vi "Model Identifyer.vi"(9 "Manufacturer":T1=enum."red", 11 "ID String":string) -> (1 "Result":bool)   [LabVIEW 2014, in "Universal Power Meter.lvlib" / "Universal Power Meter.lvclass"]
uses:
  Universal Power Meter.lvclass
  Manufacturer List.ctl
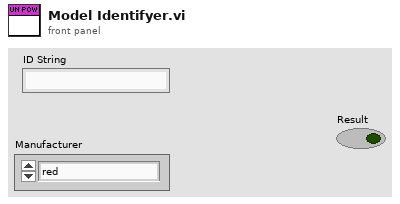
[diagram p1: front panel]
types:
  T1 = typedef "Manufacturer List.ctl" = enum16{"National Instruments", "TEKTRONIX", "FLUKE", "dummy", "red", "YOKOGAWA"}
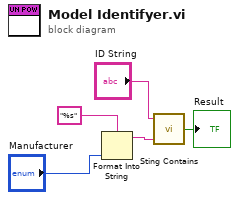
[diagram p0: block diagram]
diagram:
  n1 = Format Into String(format string="%s", "Manufacturer") -> (resulting string=w2:string)  [unwired: 2 in, 1 out]
  n2 = call "Sting Contains.vi"("Regular expression"=w2, "Input String"="ID String") -> ("Boolean"=→"Result":bool)  [unwired: 3 in]
